vi "write_waveform_to_file.vi"(8 "Waveform Array":waveform(dbl)[](array[waveform]), 10 "Path":path) -> ()   [LabVIEW 2016]
uses:
  <vilib>/Utility/file.llb/Write To Spreadsheet File (DBL).vi
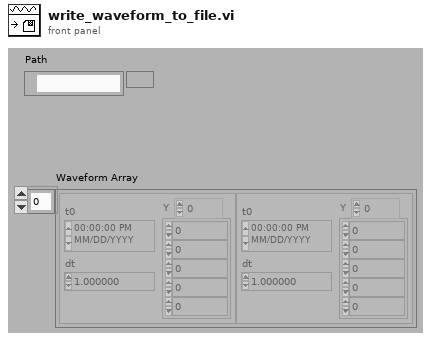
[diagram p1: front panel]
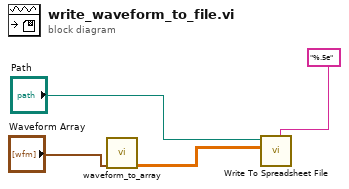
[diagram p0: block diagram]
diagram:
  n1 = call "waveform_to_array.vi"("Waveform Array"="Waveform Array") -> ("Array"=w3:dbl[][])  [unwired: 10 out]
  n2 = call-poly <vilib>:"Write To Spreadsheet File.vi"("format (%.3f)"="%.5e", "2D data"=w3, "file path (dialog if empty)"="Path") -> ()  [unwired: 3 in, 3 out]
